vi "FTW-CodeGen-Prototype.vi"(0 "REPLACE_SQLite Connection":refnum<data-value>, 2 "REPLACE_SQL Script":string, 5 "ADAPT_Data to Insert":T1(array[cluster]), 7 "REPLACE_Wrap as a Transaction":bool=TRUE, 11 "REPLACE_error in":errorcluster) -> (4 "REPLACE_SQLite Connection out":refnum<data-value>, 6 "REPLACE_SQL Debug String":string, 15 "REPLACE_error out":errorcluster)   [LabVIEW 2014, in "FTW-SQLite-Insert.xnode"]
uses:
  FTW-SQLite-Insert.xnode
  src/database/core/FTW-SQLite-Core-Structure.ctl
  src/error/FTW-ERR-ThrowError.vi
  src/error/FTW-ERR-CallChain.vi
  src/string/FTW-STR-ReplaceWhitespace.vi
  src/string/FTW-STR-Array-Delimit.vi
  src/error/FTW-ERR-Clear.vi
  src/regex/FTW-Regex-ReplaceAll.vi
panel:
  # "Inputs"
  # "Outputs"
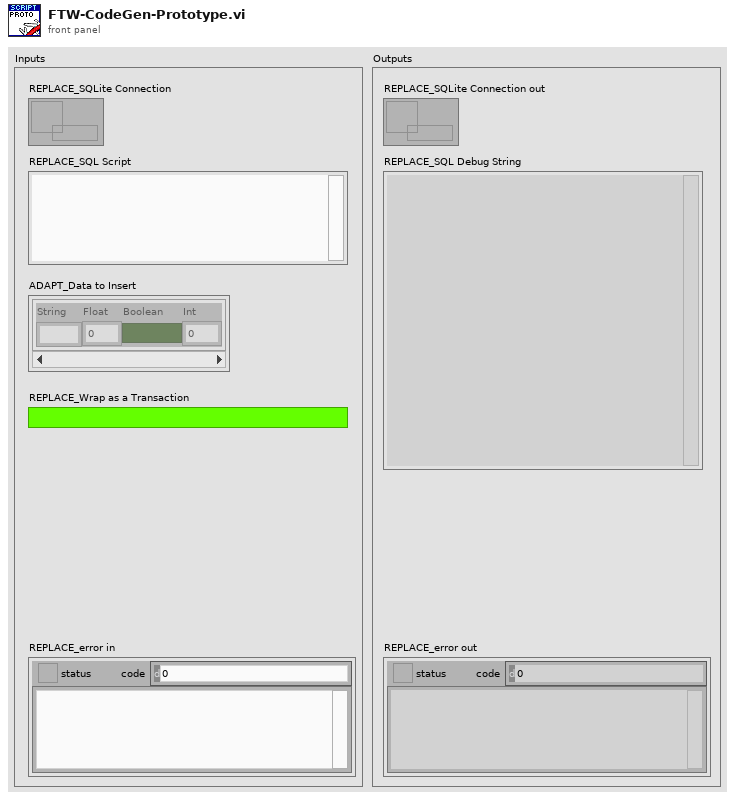
[diagram p1: front panel]
types:
  T1 = cluster{"String":string, "Float":dbl, "Boolean":bool, "Int":i64}[]
  T2 = typedef "FTW-SQLite-Core-Structure.ctl" = cluster{"Connection":u64}
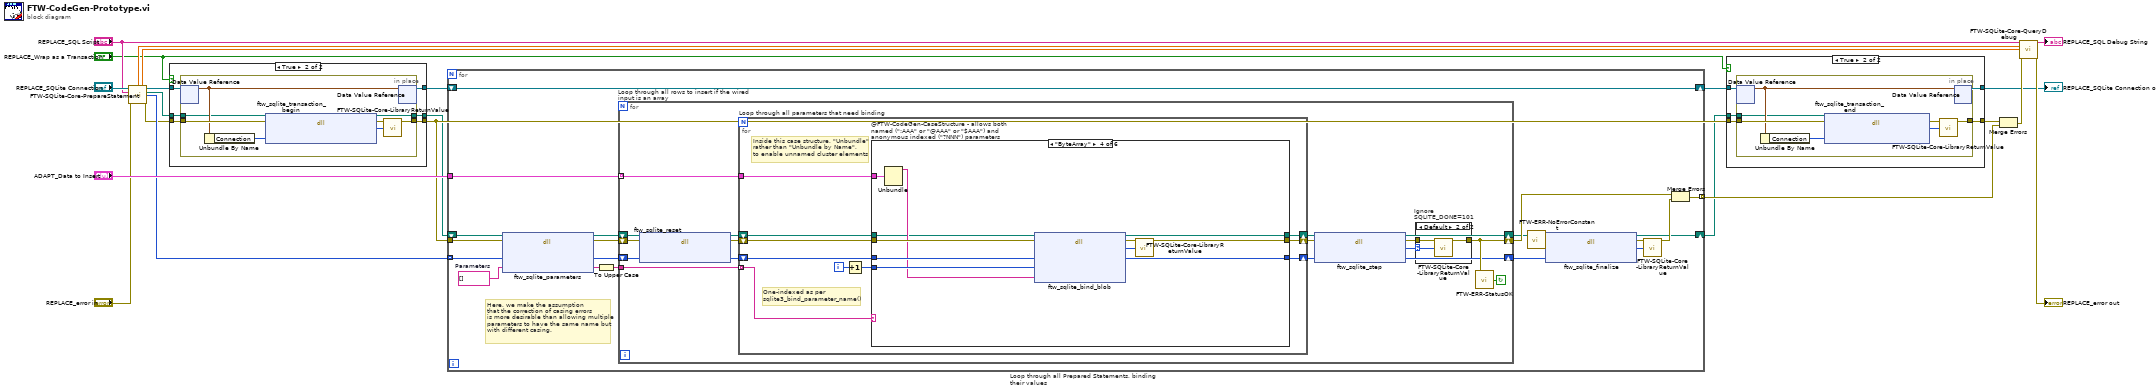
[diagram p0: block diagram]
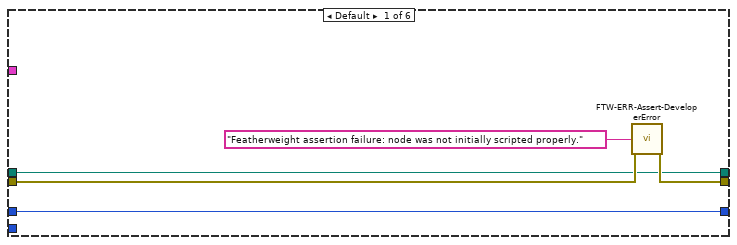
[diagram p5: hidden frame]
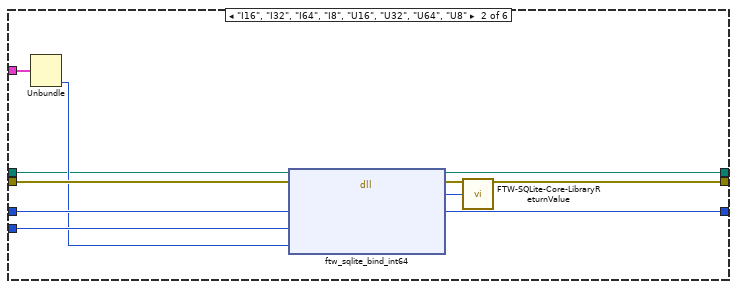
[diagram p6: hidden frame]
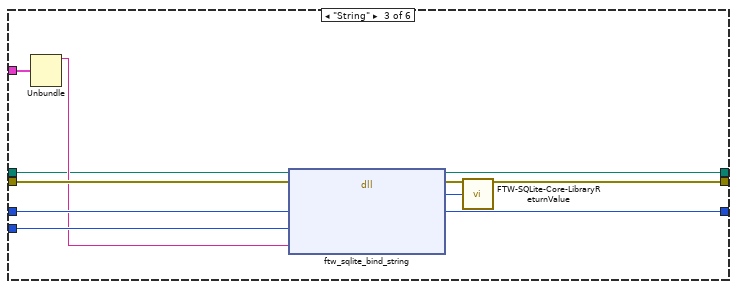
[diagram p7: hidden frame]
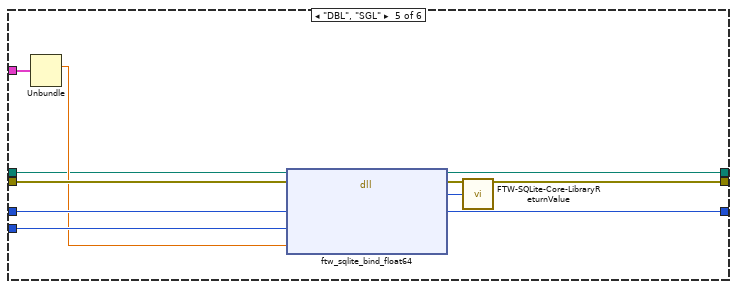
[diagram p8: hidden frame]
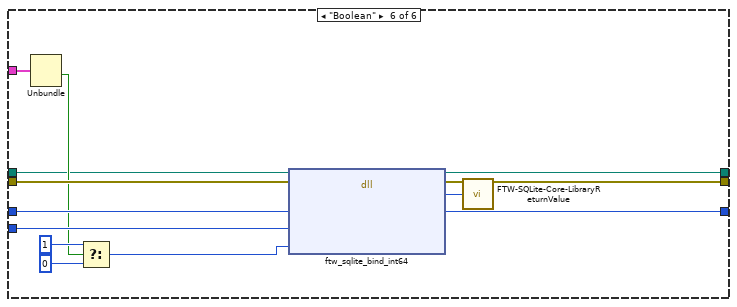
[diagram p9: hidden frame]
diagram:
  n1 = call "FTW-SQLite-Core-PrepareStatement.vi"("SQLite Connection"="REPLACE_SQLite Connection", "SQL Statement"="REPLACE_SQL Script", "error in"="REPLACE_error in") -> ("Begin Timestamp"=w15:dbl, "Compile Time"=w14:dbl, "SQLite Connection out"=w11:refnum<data-value>, "Library Filepath"=w3:path, "Prepared Statements"=w20:i64[], "error out"=w10:errorcluster)  [unwired: 7 in]
  n2 = case shown="True" "REPLACE_Wrap as a Transaction" {
    tunnel: w11 -> [w25 w31]
    tunnel: w10 -> [w24 w30]
    tunnel: [w25 w29] -> w5
    tunnel: [w24 w28] -> w8
    tunnel: w3 -> [w23 w27]
    tunnel: [w23 w26] -> w2
    frame False {
    }
    frame True {
      n3 = in-place {
        in-place-border: [w39] -> w28
        in-place-border: w30 -> [w37]
        in-place-border: w27 -> [w33]
        in-place-border: [w32] -> w26
        n4 = in-place-dvr #1(w31) -> (w36:T2)  [unwired: 1 out]
        n5 = Unbundle By Name(w36) -> ("Connection"=w38:u64)
        n6 = dll-call lib="?" fn="ftw_sqlite_transaction_begin"(path in=w33, error in=w37, "Connection Handle"=w38) -> (path out=w32:path, error out=w35:errorcluster, "Return Value"=w34:i32)  [unwired: 2 in]
        n7 = call "FTW-SQLite-Core-LibraryReturnValue.vi"("error in"=w35, "Return Value"=w34) -> ("error out"=w39:errorcluster)  [unwired: 13 in]
        n8 = in-place-dvr #1(w36) -> (w29:refnum<data-value>)  [unwired: 1 out]
      }
    }
  }
  n9 = for "Loop through all Prepared Statements, binding their values" {
    tunnel: w20 -> [w58] mode=indexing
    tunnel: "ADAPT_Data to Insert" -> [w59]
    tunnel: w8 -> [w57]
    tunnel: [w50] -> w12 mode=indexing
    shift-right: [w44] -> w4
    shift-left: w5 -> [w44]
    shift-right: [w40] -> w1
    shift-left: w2 -> [w43]
    w55 = string[] []  # Parameters
    # "Here, we make the assumption\nthat the correction of casing errors\nis more desirable than allowing multiple\nparameters to have the same name but\nwith different casing."
    n10 = dll-call lib="?" fn="ftw_sqlite_parameters"(path in=w43, error in=w57, "Prepared Statement Pointer"=w58, "Parameters to Bind"=w55) -> (path out=w42:path, error out=w56:errorcluster, "Prepared Statement Pointer"=w52:i64, "Parameters to Bind"=w54:string[])  [unwired: 2 in]
    n11 = To Upper Case(1:w54) -> (0:w53:string[])
    n12 = for "Loop through all rows to insert if the wired input is an array" {
      shift-right: [w73] -> w49
      shift-left: w56 -> [w66]
      tunnel: w59 -> [w72] mode=indexing
      tunnel: w53 -> [w69]
      shift-right: [w68] -> w51
      shift-left: w52 -> [w65]
      shift-right: [w60] -> w41
      shift-left: w42 -> [w63]
      stop <- w70 continue-if-true
      n13 = dll-call lib="?" fn="ftw_sqlite_reset"(path in=w63, error in=w66, "Prepared Statement Pointer"=w65) -> (path out=w62:path, error out=w67:errorcluster, "Prepared Statement Pointer"=w64:i64)  [unwired: 2 in]
      n14 = for "Loop through all parameters that need binding" {
        shift-right: [w89] -> w76
        shift-left: w67 -> [w86]
        shift-right: [w90] -> w75
        shift-left: w64 -> [w83]
        tunnel: w72 -> [w88]
        tunnel: w69 -> [w84] mode=indexing
        shift-right: [w81] -> w61
        shift-left: w62 -> [w82]
        i -> [w87]
        # "Inside this case structure, \"Unbundle\"\nrather than \"Unbundle by Name\",\nto enable unnamed cluster elements"
        # "One-indexed as per\nsqlite3_bind_parameter_name()"
        n15 = Increment(x=w87) -> (x+1=w85:i32)
        n16 = case "@FTW-CodeGen-CaseStructure - allows both named (\":AAA\" or \"@AAA\" or \"$AAA\") and anonymous indexed (\"?NNN\") parameters" shown="\"ByteArray\"" w84 {
          tunnel: w86 -> [w94 w105 w116 w127 w138 w152]
          tunnel: w83 -> [w95 w104 w115 w126 w137 w151]
          tunnel: [w95 w106 w117 w128 w139 w153] -> w90
          tunnel: [w93 w100 w111 w122 w133 w147] -> w89
          tunnel: w88 -> [_ w102 w113 w124 w135 w149]
          tunnel: w85 -> [_ w103 w114 w125 w136 w150]
          tunnel: w82 -> [w91 w96 w107 w118 w129 w141]
          tunnel: [w91 w97 w108 w119 w130 w140] -> w81
          frame Default {
            n17 = call "FTW-ERR-Assert-DeveloperError.vi"("Reason this error should never happen"="Featherweight assertion failure: node was not initially scripted properly.", "error in"=w94) -> ("error out"=w93:errorcluster)  [unwired: 13 in]
          }
          frame "I16", "I32", "I64", "I8", "U16", "U32", "U64", "U8" {
            n18 = Unbundle(w102) -> ("Int"=w98:i64)  [unwired: 3 out]
            n19 = dll-call lib="?" fn="ftw_sqlite_bind_int64"(path in=w96, error in=w105, "Prepared Statement Pointer"=w104, "Parameter Index"=w103, "I64 Value"=w98) -> (path out=w97:path, error out=w101:errorcluster, "Return Value"=w99:i32, "Prepared Statement Pointer"=w106:i64)  [unwired: 3 in]
            n20 = call "FTW-SQLite-Core-LibraryReturnValue.vi"("error in"=w101, "Return Value"=w99) -> ("error out"=w100:errorcluster)  [unwired: 13 in]
          }
          frame "String" {
            n21 = Unbundle(w113) -> ("String"=w109:string)  [unwired: 3 out]
            n22 = dll-call lib="?" fn="ftw_sqlite_bind_string"(path in=w107, error in=w116, "Prepared Statement Pointer"=w115, "Parameter Index"=w114, "Value"=w109) -> (path out=w108:path, error out=w112:errorcluster, "Return Value"=w110:i32, "Prepared Statement Pointer"=w117:i64)  [unwired: 3 in]
            n23 = call "FTW-SQLite-Core-LibraryReturnValue.vi"("error in"=w112, "Return Value"=w110) -> ("error out"=w111:errorcluster)  [unwired: 13 in]
          }
          frame "ByteArray" {
            n24 = Unbundle(w124) -> ("String"=w120:string)  [unwired: 3 out]
            n25 = dll-call lib="?" fn="ftw_sqlite_bind_blob"(path in=w118, error in=w127, "Prepared Statement Pointer"=w126, "Parameter Index"=w125, "Value"=w120) -> (path out=w119:path, error out=w123:errorcluster, "Return Value"=w121:i32, "Prepared Statement Pointer"=w128:i64)  [unwired: 3 in]
            n26 = call "FTW-SQLite-Core-LibraryReturnValue.vi"("error in"=w123, "Return Value"=w121) -> ("error out"=w122:errorcluster)  [unwired: 13 in]
          }
          frame "DBL", "SGL" {
            n27 = Unbundle(w135) -> ("Float"=w131:dbl)  [unwired: 3 out]
            n28 = dll-call lib="?" fn="ftw_sqlite_bind_float64"(path in=w129, error in=w138, "Prepared Statement Pointer"=w137, "Parameter Index"=w136, "DBL Value"=w131) -> (path out=w130:path, error out=w134:errorcluster, "Return Value"=w132:i32, "Prepared Statement Pointer"=w139:i64)  [unwired: 3 in]
            n29 = call "FTW-SQLite-Core-LibraryReturnValue.vi"("error in"=w134, "Return Value"=w132) -> ("error out"=w133:errorcluster)  [unwired: 13 in]
          }
          frame "Boolean" {
            n30 = Unbundle(w149) -> ("Boolean"=w142:bool)  [unwired: 3 out]
            n31 = Select(t=i64 1, s=w142, f=i64 0) -> (s? t:f=w145:i64)
            n32 = dll-call lib="?" fn="ftw_sqlite_bind_int64"(path in=w141, error in=w152, "Prepared Statement Pointer"=w151, "Parameter Index"=w150, "I64 Value"=w145) -> (path out=w140:path, error out=w148:errorcluster, "Return Value"=w146:i32, "Prepared Statement Pointer"=w153:i64)  [unwired: 3 in]
            n33 = call "FTW-SQLite-Core-LibraryReturnValue.vi"("error in"=w148, "Return Value"=w146) -> ("error out"=w147:errorcluster)  [unwired: 13 in]
          }
        }
      }
      n34 = dll-call lib="?" fn="ftw_sqlite_step"(path in=w61, error in=w76, "Prepared Statement Pointer"=w75) -> (path out=w60:path, error out=w74:errorcluster, "Return Value"=w71:i32, "Prepared Statement Pointer"=w68:i64)  [unwired: 1 in]
      n35 = case "Ignore\nSQLITE_DONE=101" shown="Default" w71 {
        selector: w71 -> [_ w78]
        tunnel: w74 -> [w77 w80]
        tunnel: [w77 w79] -> w73
        frame 101 {
        }
        frame Default {
          n36 = call "FTW-SQLite-Core-LibraryReturnValue.vi"("error in"=w80, "Return Value"=w78) -> ("error out"=w79:errorcluster)  [unwired: 13 in]
        }
      }
      n37 = call "FTW-ERR-StatusOK.vi"("error to check"=w73) -> ("Status OK?"=w70:bool)
    }
    n38 = call "FTW-ERR-NoErrorConstant.vi"() -> ("no error"=w45:errorcluster)
    n39 = dll-call lib="?" fn="ftw_sqlite_finalize"(path in=w41, error in=w45, "Prepared Statement Pointer"=w51) -> (path out=w40:path, error out=w48:errorcluster, "Return Value"=w46:i32)  [unwired: 2 in]
    n40 = call "FTW-SQLite-Core-LibraryReturnValue.vi"("error in"=w48, "Return Value"=w46) -> ("error out"=w47:errorcluster)  [unwired: 13 in]
    n41 = Merge Errors(w49, w47) -> (w50:errorcluster)
  }
  n42 = case shown="True" "REPLACE_Wrap as a Transaction" {
    tunnel: w4 -> [w155 w160]
    tunnel: [w155 w159] -> w9
    tunnel: w8 -> [w154 w158]
    tunnel: [w154 w157] -> w7
    tunnel: w1 -> [_ w156]
    frame False {
    }
    frame True {
      n43 = in-place {
        in-place-border: [w167] -> w157
        in-place-border: w158 -> [w165]
        in-place-border: w156 -> [w161]
        n44 = in-place-dvr #2(w160) -> (w164:T2)  [unwired: 1 out]
        n45 = Unbundle By Name(w164) -> ("Connection"=w166:u64)
        n46 = dll-call lib="?" fn="ftw_sqlite_transaction_end"(path in=w161, error in=w165, "Connection Handle"=w166) -> (error out=w163:errorcluster, "Return Value"=w162:i32)  [unwired: 2 in, 1 out]
        n47 = call "FTW-SQLite-Core-LibraryReturnValue.vi"("error in"=w163, "Return Value"=w162) -> ("error out"=w167:errorcluster)  [unwired: 13 in]
        n48 = in-place-dvr #2(w164) -> (w159:refnum<data-value>)  [unwired: 1 out]
      }
    }
  }
  "REPLACE_SQLite Connection out" <- w9
  n49 = Merge Errors(w7, w12) -> (w13:errorcluster)
  n50 = call "FTW-SQLite-Core-QueryDebug.vi"("SQL Script"="REPLACE_SQL Script", "Begin Timestamp"=w15, "Compile Time"=w14, "error in"=w13) -> ("SQL Debug String"=→"REPLACE_SQL Debug String":string, "error out"=→"REPLACE_error out":errorcluster)  [unwired: 10 in]
